vi "LAS-CTS_SingleSpotMonitor.vi"() -> ()   [LabVIEW 2024]
uses:
  <vilib>/httpClient/LabVIEWHTTPClient.lvlib
  <vilib>/Analysis/NI_AALBase.lvlib
  <vilib>/Analysis/baseanly.llb/Mean (DBL).vi
panel:
  out "last file name":string
  out "standard deviation":dbl format="%0.2f"
  out "mean":dbl format="%0.2f"
  in  "base filename":string
  in  "file number":i32 format="%03d"
  out "Waveform Chart":dbl(graph)
  in  "Post-read delay (ms)":u32
  out "# of laser readings":i32
  in  "Z position (mirror mm)":string
  in  "X position (mirror mm)":string
  in  "Target ID":string
  in  "data filepath":path
  in  "Number of Pulses":i32
  out "Laser On/Off":bool
  out "Pulses Remaining":i32
  out "Laser Energy (uJ)":dbl format="%#.3f"
  in  "# data points":i32
  in  "Energy Meter":refnum<visa-resource-name>
  in  "Keithly":refnum<visa-resource-name>
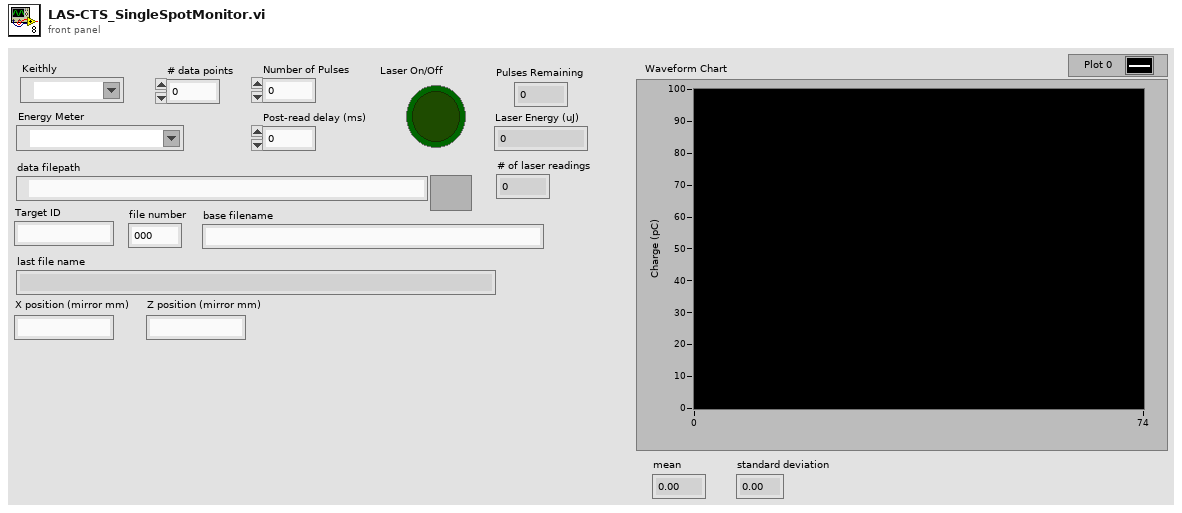
[diagram p1: front panel]
types:
  T1 = enum16{"open", "replace", "create", "open or create", "replace or create", "replace or create with confirmation"}
  T2 = typedef "LabVIEWHTTPClient.lvlib/ClientHandle.ctl" = refnum<k1>
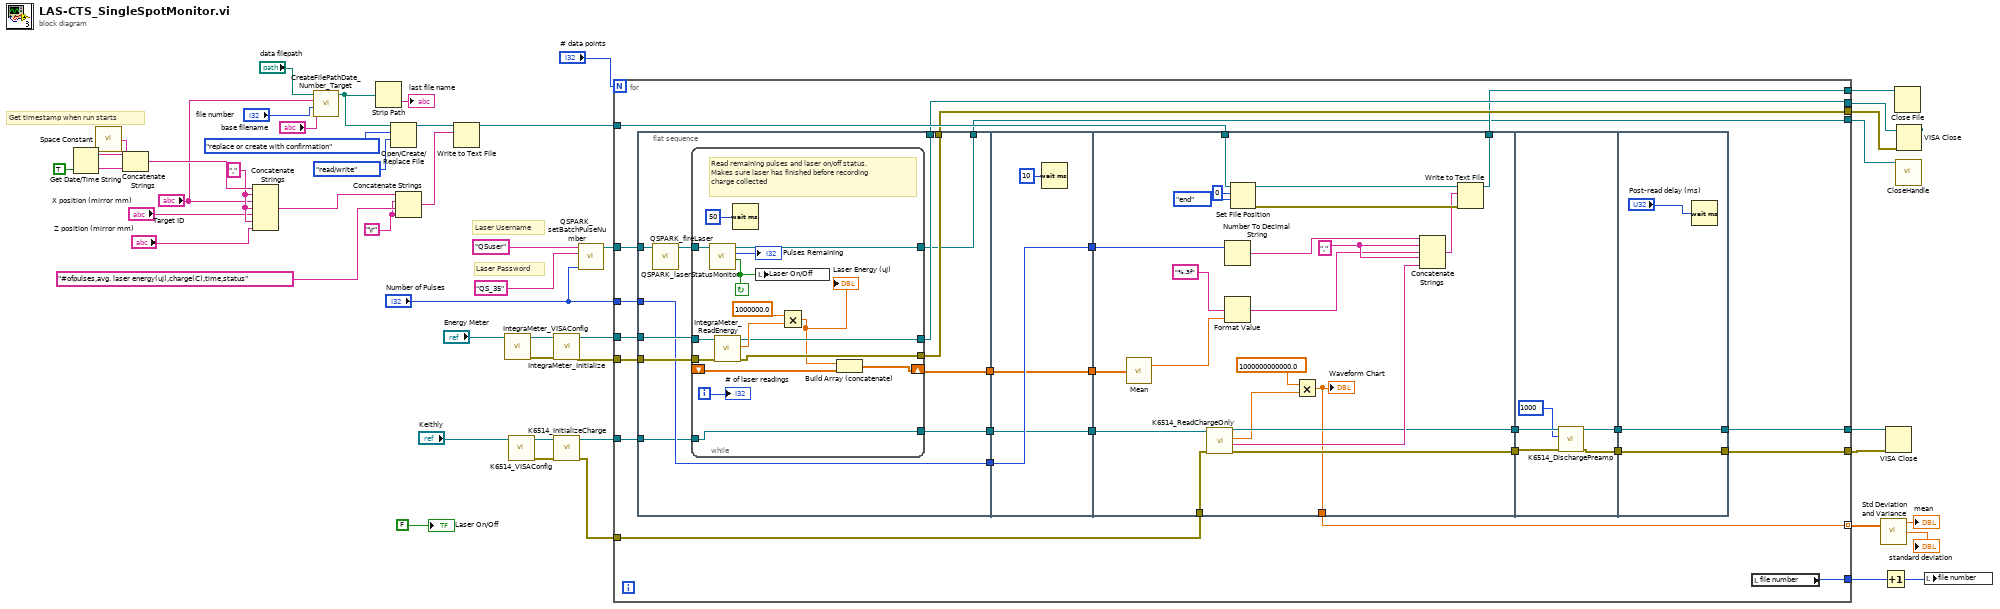
[diagram p0: block diagram]
diagram:
  w16 = "," ("string")
  w30 = "\r"
  # "Get timestamp when run starts"
  # "Laser Password"
  # "Laser Username"
  n1 = Get Date/Time String(want seconds? (F)=TRUE) -> (date string=w29:string, time string=w28:string)  [unwired: 2 in]
  n2 = call <vilib>:"Space Constant.vi"() -> ("String"=w27:string)
  n3 = Concatenate Strings(w29, w27, w28) -> (w25:string)
  n4 = Concatenate Strings(w25, w16, "Target ID", w16, "X position (mirror mm)", w16, "Z position (mirror mm)") -> (w24:string)
  n5 = call "CreateFilePathDate_Number_Target.vi"("base filename"="base filename", "file number"="file number", "Target ID"="Target ID", "data filepath"="data filepath") -> ("appended path"=w3:path)  [unwired: 7 in]
  n6 = Strip Path(path=w3) -> (name=→"last file name":string)  [unwired: 1 out]
  n7 = Open/Create/Replace File(file path (use dialog)=w3, operation (0:open)=T1."replace or create with confirmation", access (0:read/write)=enum16{"read/write", "read-only", "write-only"}."read/write") -> (refnum out=w33:refnum<file>)  [unwired: 3 in, 2 out]
  n8 = Concatenate Strings(w24, w30, "#ofpulses,avg. laser energy(uJ),charge(C),time,status", w30) -> (w31:string)
  n9 = Write to Text File(file (use dialog)=w33, text=w31) -> (refnum out=w23:refnum<file>)  [unwired: 2 in, 2 out]
  n10 = call "IntegraMeter_VISAConfig.vi"("VISA resource name"="Energy Meter") -> ("error out"=w46:errorcluster, "reference out"=w45:refnum<visa-resource-name>)  [unwired: 9 in]
  n11 = call "K6514_VISAConfig.vi"("VISA resource name"="Keithly") -> ("error out"=w49:errorcluster, "reference out"=w48:refnum<visa-resource-name>)  [unwired: 9 in]
  n12 = call "IntegraMeter_Initialize.vi"("error in"=w46, "VISA resource name"=w45) -> ("error out"=w41:errorcluster, "VISA resource name out"=w42:refnum<visa-resource-name>)  [unwired: 8 in]
  n13 = call "K6514_InitializeCharge.vi"("error in (no error)"=w49, "VISA resource name"=w48) -> ("error out"=w36:errorcluster, "VISA resource name out"=w1:refnum<visa-resource-name>)  [unwired: 8 in]
  n14 = call "QSPARK_setBatchPulseNumber.vi"("Number of Pulses"="Number of Pulses", "password"="QS_35", "username"="QSuser") -> ("client handle out"=w38:T2)  [unwired: 8 in]
  n15 = for {
    N: "# data points" -> [_]
    tunnel: w42 -> [w74]
    tunnel: w41 -> [w73]
    tunnel: w38 -> [w72]
    tunnel: w36 -> [w71]
    tunnel: w23 -> [w68]
    tunnel: [w67] -> w22
    tunnel: [w66] -> w21
    tunnel: [w65] -> w20
    tunnel: [w64] -> w19
    tunnel: [w63] -> w18
    tunnel: [w62] -> w17
    tunnel: "Number of Pulses" -> [w59]
    tunnel: [w54] -> w8 mode=indexing
    tunnel: [w53] -> w4
    tunnel: w1 -> [w52]
    n16 = flat-sequence {
      tunnel: w74 -> [w85]
      tunnel: w73 -> [w84]
      tunnel: w72 -> [w82]
      tunnel: [w81] -> w65
      tunnel: [w80] -> w64
      tunnel: [w79] -> w62
      tunnel: [w78] -> w60
      tunnel: w59 -> [w78]
      tunnel: [w77] -> w56
      tunnel: w52 -> [w76]
      tunnel: [w75] -> w50
      tunnel: [w104] -> w61
      tunnel: w60 -> [w104]
      tunnel: w56 -> [w103]
      tunnel: [w103] -> w55
      tunnel: [w102] -> w51
      tunnel: w50 -> [w102]
      tunnel: w71 -> [w118]
      tunnel: [w116] -> w70
      tunnel: [w115] -> w69
      tunnel: w68 -> [w114]
      tunnel: [w113] -> w63
      tunnel: w61 -> [w112]
      tunnel: w55 -> [w109]
      tunnel: [w107] -> w54
      tunnel: w51 -> [w106]
      tunnel: w70 -> [w132]
      tunnel: w69 -> [w131]
      tunnel: [w129] -> w58
      tunnel: [w128] -> w57
      tunnel: [w134] -> w66
      tunnel: [w135] -> w67
      tunnel: w58 -> [w135]
      tunnel: w57 -> [w134]
      frame #0 {
        n17 = call "QSPARK_fireLaser.vi"("client handle"=w82) -> ("client handle out"=w83:T2)  [unwired: 10 in]
        n18 = while {
          tunnel: w83 -> [w100]
          tunnel: [w99] -> w79
          shift-right: [w93] -> w77
          shift-left: _ -> [w96]
          tunnel: w85 -> [w92]
          tunnel: w84 -> [w91]
          tunnel: [w90] -> w81
          tunnel: [w89] -> w80
          tunnel: w76 -> [w86]
          tunnel: [w86] -> w75
          i -> [w88]
          stop <- w97 continue-if-true
          # "Read remaining pulses and laser on/off status. \nMakes sure laser has finished before recording \ncharge collected"
          n19 = call "QSPARK_laserStatusMonitor.vi"("client handle"=w100) -> ("laser on?"=w97:bool, "remaining pulses"=→"Pulses Remaining":i32, "client handle out"=w99:T2)  [unwired: 8 in]
          n20 = call "IntegraMeter_ReadEnergy.vi"("error in (no error)"=w91, "VISA resource name"=w92) -> ("error out"=w89:errorcluster, "Laser Energy (J)"=w94:dbl, "VISA resource name out"=w90:refnum<visa-resource-name>)  [unwired: 7 in]
          n21 = Wait (ms)(milliseconds to wait=u32 50 ("millisecond multiple")) -> ()  [unwired: 1 out]
          n22 = local write "Laser On/Off"(w97) -> ()
          n23 = Multiply(x=1000000.0, y=w94) -> (x*y=w87:dbl)
          "Laser Energy (uJ)" <- w87
          n24 = Build Array (concatenate)(w87, w96) -> (w93:dbl[])
          "# of laser readings" <- w88
        }
      }
      frame #1 {
        n25 = Wait (ms)(milliseconds to wait=u32 10) -> ()  [unwired: 1 out]
      }
      frame #2 {
        w121 = "," ("string")
        n26 = call-poly <vilib>:"Mean.vi"("X"=w109) -> ("mean"=w108:dbl)  [unwired: 1 out]
        n27 = call "K6514_ReadChargeOnly.vi"("error in (no error)"=w118, "VISA resource name"=w106) -> ("error out"=w116:errorcluster, "Response"=w117:string, "charge(C)"=w111:dbl, "VISA resource name out"=w115:refnum<visa-resource-name>)  [unwired: 5 in]
        n28 = Number To Decimal String(number=w112) -> (decimal integer string=w122:string)  [unwired: 1 in]
        n29 = Format Value(format string="%.3f", value (0)=w108) -> (output string=w119:string)  [unwired: 1 in]
        n30 = Set File Position(offset (in bytes) (0)=i64 0, refnum=w114, from (0:start)=enum16{"start", "end", "current"}."end") -> (refnum out=w124:refnum<file>, error out=w127:errorcluster)  [unwired: 1 in]
        n31 = Multiply(x=1000000000000.0, y=w111) -> (x*y=w107:dbl)
        "Waveform Chart" <- w107
        n32 = Concatenate Strings(w122, w121, w119, w121, w117) -> (w123:string)
        n33 = Write to Text File(file (use dialog)=w124, text=w123, error in=w127) -> (refnum out=w113:refnum<file>)  [unwired: 1 in, 2 out]
      }
      frame #3 {
        n34 = call "K6514_DischargePreamp.vi"("error in (no error)"=w132, "discharge time (ms)"=1000, "VISA resource name in"=w131) -> ("error out"=w128:errorcluster, "VISA resource name out"=w129:refnum<visa-resource-name>)  [unwired: 7 in]
      }
      frame #4 {
        n35 = Wait (ms)(milliseconds to wait="Post-read delay (ms)") -> ()  [unwired: 1 out]
      }
    }
    n36 = local read "file number"() -> (w53:i32)
  }
  n37 = call <vilib>:"Std Deviation and Variance.vi"("X"=w8) -> ("mean"=→"mean":dbl, "standard deviation"=→"standard deviation":dbl)  [unwired: 1 in, 1 out]
  n38 = Increment(x=w4) -> (x+1=w5:i32)
  n39 = VISA Close(VISA resource name=w22, error in (no error)=w21) -> ()  [unwired: 1 out]
  n40 = Close File(refnum=w18) -> ()  [unwired: 1 in, 2 out]
  n41 = call <vilib>:"CloseHandle.vi"("client handle"=w17) -> ()  [unwired: 14 in, 1 out]
  n42 = VISA Close(VISA resource name=w20, error in (no error)=w19) -> ()  [unwired: 1 out]
  n43 = local write "file number"(w5) -> ()
  "Laser On/Off" <- FALSE ("Laser On/Off")
